vi "Actor Core.vi"(8 "error in":errorcluster, 11 "My Application":refnum<class "Actor Template.lvclass">) -> (0 "error out":errorcluster, 3 "Actor out":refnum<class "Actor.lvclass">)   [LabVIEW 2012, in "Actor Template.lvlib" / "Actor Template.lvclass"]
doc: "This is Actor Core.vi, the main message handling loop for Actors. An actor usually just sits in this loop and processes messages as they arrive. Any error returned by the message Do.vi call will stop the loop, with error code 43 as the canonical signal to stop with no error sent to caller. Descendants may override that in Handle Error.vi."
uses:
  Actor Template.lvclass
  <vilib>/ActorFramework/Actor/Actor.lvclass
  Aquire Data Actor/Aquire Data/Aquire Data.lvclass
  Display Data Actor/Display Data/Display Data.lvclass
  <vilib>/ActorFramework/Actor/Actor.lvclass/Actor.ctl
  <vilib>/ActorFramework/Message Enqueuer/Message Enqueuer.lvclass/Message Enqueuer.ctl
  Actor Template.lvclass/Actor Template.ctl
  Aquire Data Actor/Aquire Data Task Msg/Aquire Data Task Msg.lvclass/Aquire Data Task Msg.ctl
  Display Data Actor/Display Data Task Msg/Display Data Task Msg.lvclass/Display Data Task Msg.ctl
  <vilib>/ActorFramework/Message Enqueuer/Init from Existing Queue.vi
  <vilib>/ActorFramework/Message Enqueuer/Enqueue.vi
  <vilib>/ActorFramework/Message Priority Queue/Priority Enqueue.vi
  <vilib>/ActorFramework/Message Enqueuer/Message Enqueuer.lvclass
  <vilib>/ActorFramework/Stop Msg/Stop Msg.lvclass
  Aquire Data Actor/Aquire Data Task Msg/Aquire Data Task Msg.lvclass
  Display Data Actor/Display Data Task Msg/Display Data Task Msg.lvclass
panel:
  in  "stop signal":bool
  out "Event Log":string
  in  "DNL_Stop":bool
  in  "Message to Display Data":bool
  in  "Message to Aquire Data":bool
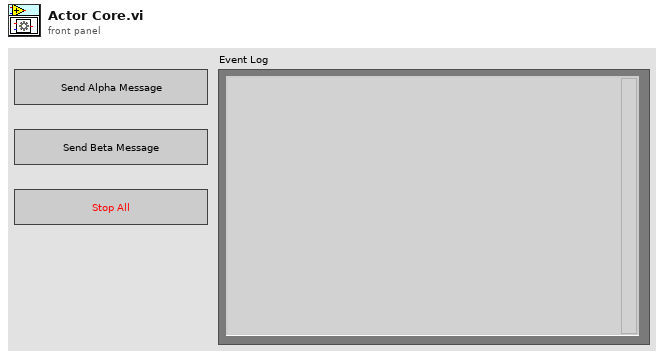
[diagram p1: front panel]
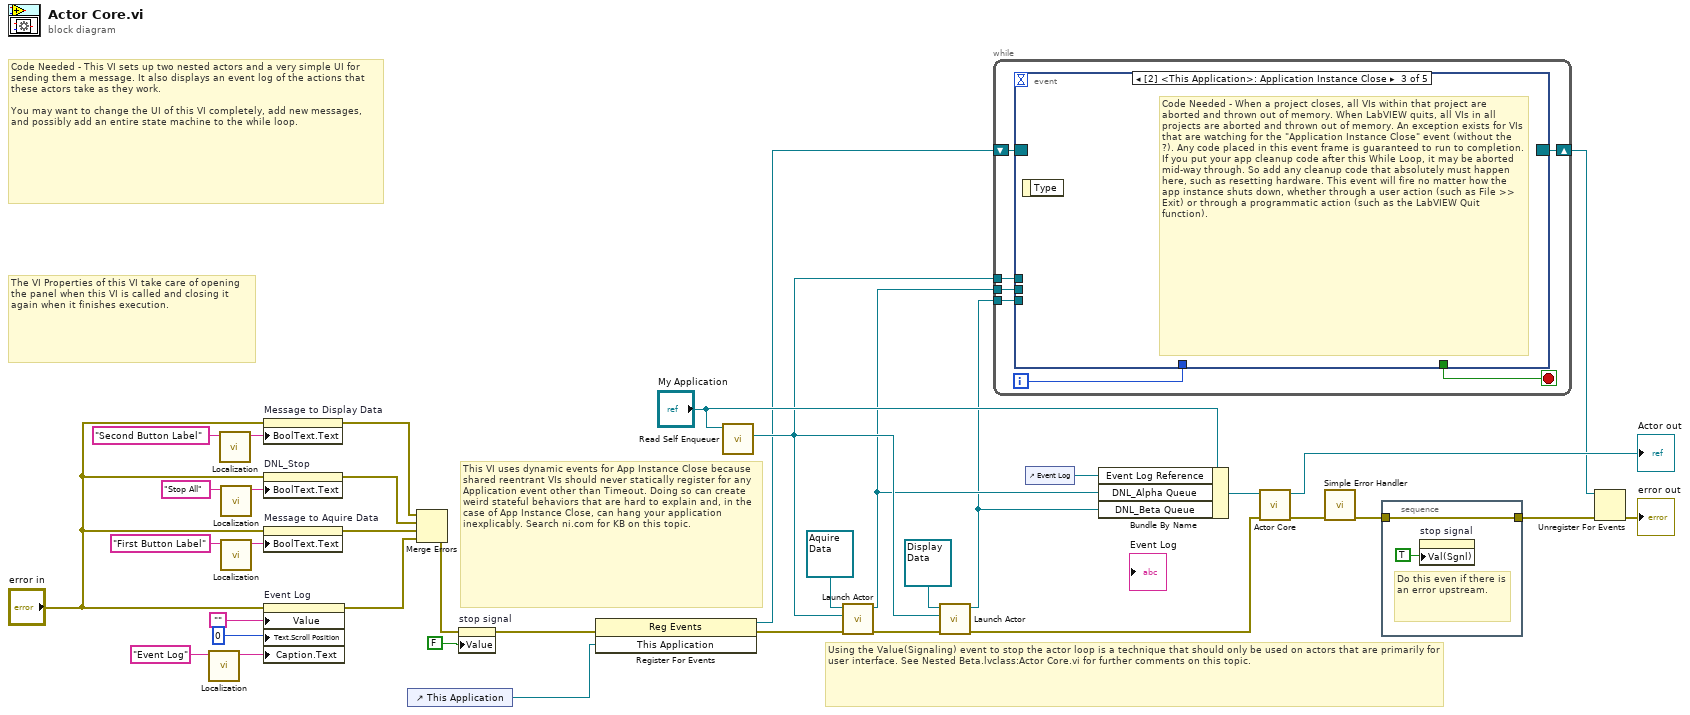
[diagram p0: block diagram]
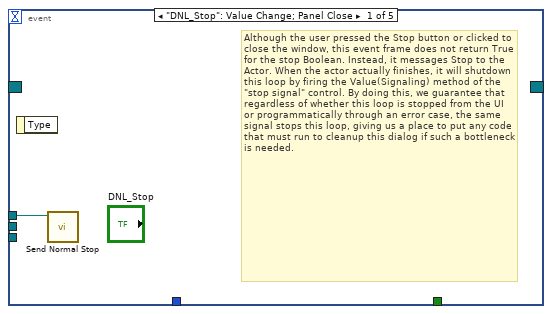
[diagram p2: hidden frame]
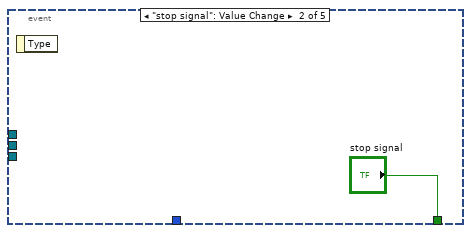
[diagram p3: hidden frame]
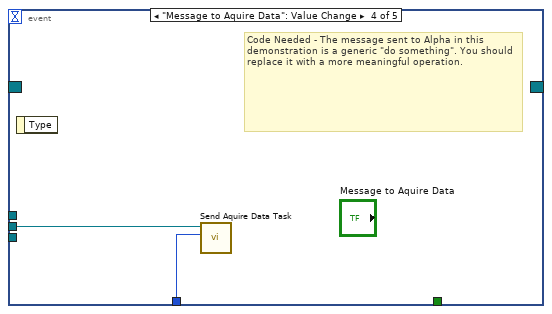
[diagram p4: hidden frame]
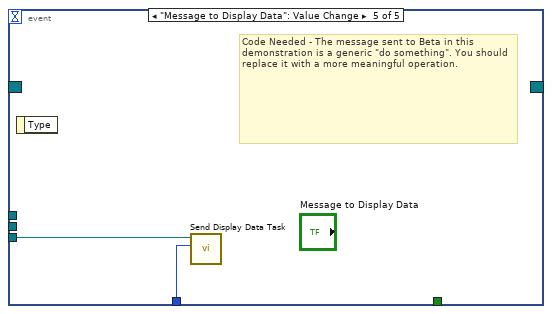
[diagram p5: hidden frame]
diagram:
  # "This VI uses dynamic events for App Instance Close because shared reentrant VIs should never statically register for any Application event other than Timeout. Doing so can create weird stateful behaviors that are hard to explain and, in the case of App Instance Close, can hang your application inexplicably. Search ni.com for KB on this topic."
  # "The VI Properties of this VI take care of opening the panel when this VI is called and closing it again when it finishes execution."
  # "Using the Value(Signaling) event to stop the actor loop is a technique that should only be used on actors that are primarily for user interface. See Nested Beta.lvclass:Actor Core.vi for further comments on this topic."
  # "Code Needed - This VI sets up two nested actors and a very simple UI for sending them a message. It also displays an event log of the actions that these actors take as they work. \n\nYou may want to change the UI of this VI completely, add new messages, and possibly add an entire state machine to the while loop."
  n1 = call "Localization.vi"("Unlocalized"="Event Log") -> ("Localized"=w21:string)  [unwired: 10 in]
  n2 = call "Localization.vi"("Unlocalized"="Second Button Label") -> ("Localized"=w15:string)  [unwired: 10 in]
  n3 = call "Localization.vi"("Unlocalized"="Stop All") -> ("Localized"=w17:string)  [unwired: 10 in]
  n4 = call "Localization.vi"("Unlocalized"="First Button Label") -> ("Localized"=w19:string)  [unwired: 10 in]
  n5 = property on="Message to Display Data" class="Bool"(error in="error in", "BoolText.Text"=w15) -> (error out=w14:errorcluster)  [unwired: 1 in, 1 out]
  n6 = property on="DNL_Stop" class="Bool"(error in="error in", "BoolText.Text"=w17) -> (error out=w13:errorcluster)  [unwired: 1 in, 1 out]
  n7 = property on="Message to Aquire Data" class="Bool"(error in="error in", "BoolText.Text"=w19) -> (error out=w12:errorcluster)  [unwired: 1 in, 1 out]
  n8 = property on="Event Log" class="Str"(error in="error in", "Value"="", "Text.Scroll Position"=u32 0, "Caption.Text"=w21) -> (error out=w11:errorcluster)  [unwired: 1 in, 1 out]
  n9 = control-ref of="This Application"() -> (w1:refnum<vi>)
  n10 = Merge Errors(w14, w13, w12, w11) -> (w10:errorcluster)
  n11 = property on="stop signal" class="Bool (strict)"(error in=w10, "Value"=FALSE ("stop")) -> (error out=w3:errorcluster)  [unwired: 1 in, 1 out]
  n12 = register-events(error in=w3, w1) -> (reference out=w7:refnum<event-registration>, error out=w2:errorcluster)  [unwired: 1 in]
  n13 = call <vilib>:"Read Self Enqueuer.vi"("Actor"="My Application") -> ("Self Enqueuer"=w29:refnum<class "Message Enqueuer.lvclass">)  [unwired: 10 in]
  n14 = call <vilib>:"Launch Actor.vi"("error in (no error)"=w2, "Actor-to-Caller Enqueuer"=w29, "Actor"=refnum<class "Aquire Data.lvclass"> refnum ("Alpha.lvclass")) -> ("error out"=w34:errorcluster, "Caller-To-Actor Enqueuer"=w28:refnum<class "Message Enqueuer.lvclass">)  [unwired: 7 in]
  n15 = call <vilib>:"Launch Actor.vi"("error in (no error)"=w34, "Actor-to-Caller Enqueuer"=w29, "Actor"=refnum<class "Display Data.lvclass"> refnum ("Beta.lvclass")) -> ("error out"=w33:errorcluster, "Caller-To-Actor Enqueuer"=w27:refnum<class "Message Enqueuer.lvclass">)  [unwired: 7 in]
  n16 = while {
    tunnel: w29 -> [w44]
    tunnel: w28 -> [w43]
    tunnel: w27 -> [w42]
    shift-right: [w38] -> w6
    shift-left: w7 -> [w39]
    i -> [w40]
    stop <- w41 stop-if-true
    n17 = event shown="[2] <This Application>: Application Instance Close" {
      selector: w39 -> [_ _ _ _ _]
      dyn-events: [_ _ _ _ _] -> w38
      timeout: _ -> [_ _ _ _ _]
      tunnel: w44 -> [w45 _ _ _ _]
      tunnel: w43 -> [_ _ _ w48 _]
      tunnel: w42 -> [_ _ _ _ w50]
      tunnel: [_ "stop signal" _ _ _] -> w41
      tunnel: w40 -> [_ _ _ w47 w49]
      event "DNL_Stop": Value Change; Panel Close {
        # "Although the user pressed the Stop button or clicked to close the window, this event frame does not return True for the stop Boolean. Instead, it messages Stop to the Actor. When the actor actually finishes, it will shutdown this loop by firing the Value(Signaling) method of the \"stop signal\" control. By doing this, we guarantee that regardless of whether this loop is stopped from the UI or programmatically through an error case, the same signal stops this loop, giving us a place to put any code that must run to cleanup this dialog if such a bottleneck is needed."
        n18 = event-data() -> ()  [unwired: 1 in, 1 out]
        n19 = call <vilib>:"Send Normal Stop.vi"("Message Enqueuer"=w45) -> ()  [unwired: 10 in, 1 out]
      }
      event "stop signal": Value Change {
        n20 = event-data() -> ()  [unwired: 1 in, 1 out]
      }
      event Application Instance Close {
        # "Code Needed - When a project closes, all VIs within that project are aborted and thrown out of memory. When LabVIEW quits, all VIs in all projects are aborted and thrown out of memory. An exception exists for VIs that are watching for the \"Application Instance Close\" event (without the ?). Any code placed in this event frame is guaranteed to run to completion. If you put your app cleanup code after this While Loop, it may be aborted mid-way through. So add any cleanup code that absolutely must happen here, such as resetting hardware. This event will fire no matter how the app instance shuts down, whether through a user action (such as File >> Exit) or through a programmatic action (such as the LabVIEW Quit function)."
        n21 = event-data() -> ()  [unwired: 1 in, 1 out]
      }
      event "Message to Aquire Data": Value Change {
        # "Code Needed - The message sent to Alpha in this demonstration is a generic \"do something\". You should replace it with a more meaningful operation."
        n22 = event-data() -> ()  [unwired: 1 in, 1 out]
        n23 = call "Send Aquire Data Task.vi"("Data"=w47, "Message Enqueuer"=w48) -> ()  [unwired: 9 in, 1 out]
      }
      event "Message to Display Data": Value Change {
        # "Code Needed - The message sent to Beta in this demonstration is a generic \"do something\". You should replace it with a more meaningful operation."
        n24 = event-data() -> ()  [unwired: 1 in, 1 out]
        n25 = call "Send Display Data Task.vi"("Data"=w49, "Message Enqueuer"=w50) -> ()  [unwired: 9 in, 1 out]
      }
    }
  }
  n26 = control-ref of="Event Log"() -> (w30:refnum<vi>)
  n27 = Bundle By Name(cluster="My Application", "Event Log Reference"=w30, "DNL_Alpha Queue"=w28, "DNL_Beta Queue"=w27) -> (w31:refnum<class "Actor Template.lvclass">)
  n28 = call-parent "Actor Core.vi"("error in"=w33, "Actor in"=w31) -> ("error out"=w9:errorcluster, "Actor out"=→"Actor out":refnum<class "Actor.lvclass">)  [unwired: 8 in]
  n29 = call <vilib>:"Simple Error Handler.vi"("error in (no error)"=w9) -> ("error out"=w8:errorcluster)  [unwired: 4 in, 4 out]
  n30 = stacked-sequence {
    tunnel: [w51] -> w5
    tunnel: w8 -> [w51]
    frame #0 {
      # "Do this even if there is an error upstream."
      n31 = property on="stop signal" class="Bool (strict)"("Val(Sgnl)"=TRUE ("stop")) -> ()  [unwired: 2 in, 2 out]
    }
  }
  n32 = Unregister For Events(event registration refnum=w6, error in=w5) -> (error out=→"error out":errorcluster)
